vi "ForLoop-Ver2.vi"() -> ()   [LabVIEW 2018]
panel:
  in  "Start Loop":bool
  out "For Loop Output":string
  # "Start Loop"
  # "Stop Loop"
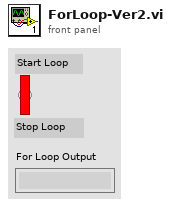
[diagram p1: front panel]
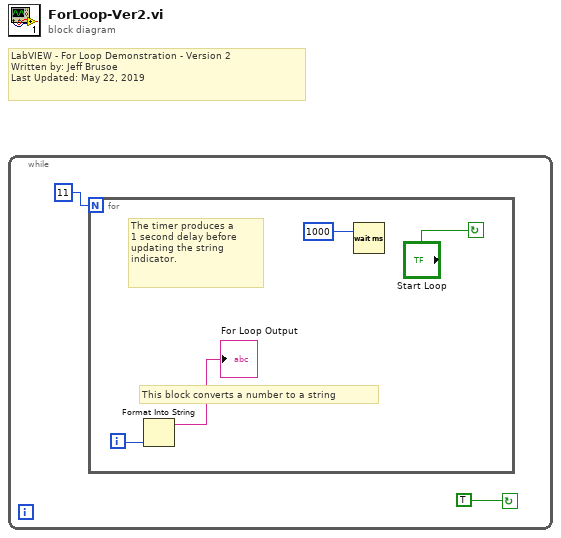
[diagram p0: block diagram]
diagram:
  # "LabVIEW - For Loop Demonstration - Version 2\nWritten by: Jeff Brusoe\nLast Updated: May 22, 2019"
  n1 = while {
    stop <- TRUE continue-if-true
    n2 = for {
      N: 11 -> [_]
      i -> [w5]
      stop <- "Start Loop" continue-if-true
      # "The timer produces a\n1 second delay before\nupdating the string\nindicator."
      # "This block converts a number to a string"
      n3 = Format Into String(w5) -> (resulting string=→"For Loop Output":string)  [unwired: 3 in, 1 out]
      n4 = Wait (ms)(milliseconds to wait=u32 1000 ("millisecond timer value")) -> ()  [unwired: 1 out]
    }
  }
